vi "Resolve Header.vi"(6 "Metadata":variant, 8 "error in (no error)":errorcluster, 11 "CubeLogger in":refnum<class "CubeLogger.lvclass">) -> (0 "error out":errorcluster, 3 "CubeLogger out":refnum<class "CubeLogger.lvclass">)   [LabVIEW 2018, in "CubeLogger.lvclass"]
uses:
  CubeLogger.lvclass
  Header.ctl
  CubeLogger.lvclass/CubeLogger.ctl
panel:
  out "Canceled?":bool
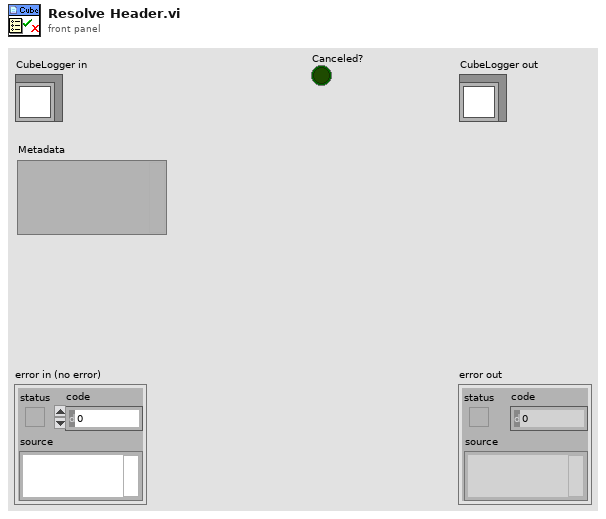
[diagram p1: front panel]
types:
  T1 = typedef "CubeLogger.lvclass/Header.ctl" = cluster{"name":string, "desc":string, "data":variant[], "meta":variant}
  T2 = enum16{"open", "replace", "create", "open or create", "replace or create", "replace or create with confirmation"}
  T3 = typedef "CubeLogger.lvclass/Dataset.ctl" = cluster{"name":string, "path":string, "size":i32[], "type":enum16{"single", "double", "uint8", "uint16", "uint32", "uint64", "int8", "int16", "int32", "int64"}, "mfmt":string}
  T4 = enum16{"single", "double", "uint8", "uint16", "uint32", "uint64", "int8", "int16", "int32", "int64"}
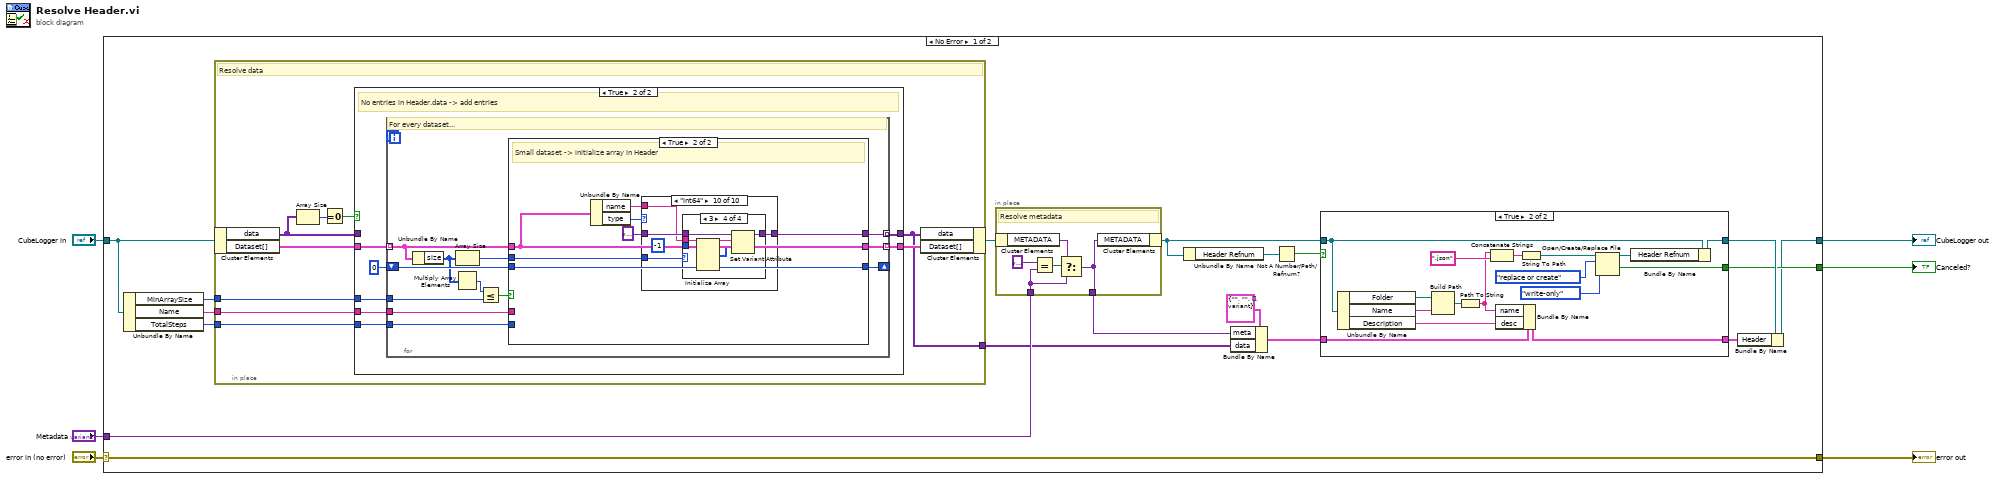
[diagram p0: block diagram]
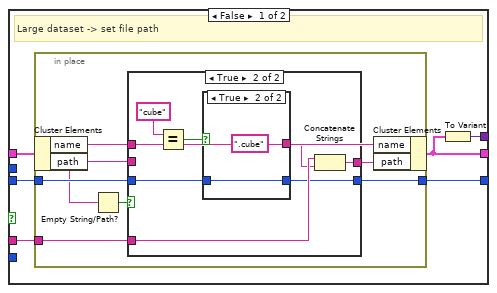
[diagram p4: hidden frame]
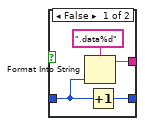
[diagram p6: hidden frame]
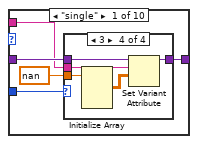
[diagram p7: hidden frame]
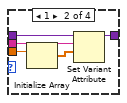
[diagram p9: hidden frame]
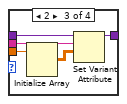
[diagram p10: hidden frame]
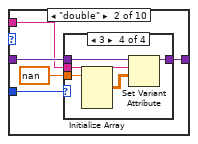
[diagram p11: hidden frame]
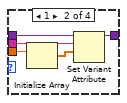
[diagram p13: hidden frame]
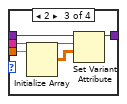
[diagram p14: hidden frame]
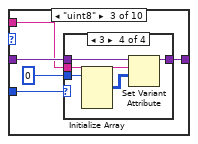
[diagram p15: hidden frame]
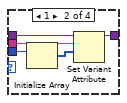
[diagram p17: hidden frame]
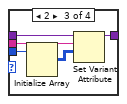
[diagram p18: hidden frame]
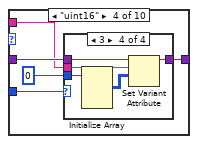
[diagram p19: hidden frame]
diagram:
  n1 = case shown="No Error" "error in (no error)" {
    selector: "error in (no error)" -> [w21 w326]
    tunnel: [w21 w326] -> w5
    tunnel: [w8 w325] -> w3
    tunnel: "CubeLogger in" -> [w23 w325]
    tunnel: "Metadata" -> [w24 _]
    tunnel: [w9 TRUE] -> w1
    frame No Error {
      n2 = Unbundle By Name(w23) -> ("MinArraySize"=w20:i32, "Name"=w19:string, "TotalSteps"=w18:i32)
      n3 = in-place {
        in-place-border: w20 -> [w49]
        in-place-border: w19 -> [w48]
        in-place-border: w18 -> [w47]
        in-place-border: [w46] -> w12
        # "Resolve data"
        n4 = in-place-cluster #1(w23) -> ("data"=w45:variant[], "Dataset[]"=w51:T3[])
        n5 = Array Size(array=w45) -> (size(s)=w44:i32)
        n6 = Equal To 0?(x=w44) -> (x = 0?=w43:bool)
        n7 = case shown="True" w43 {
          tunnel: w51 -> [w52 w60]
          tunnel: [w52 w59] -> w50
          tunnel: w49 -> [_ w58]
          tunnel: w45 -> [w53 _]
          tunnel: w48 -> [_ w57]
          tunnel: w47 -> [_ w56]
          tunnel: [w53 w55] -> w46
          frame False {
            # "Maybe: double check that everything is all right?\n   ... or not ..."
            # "Header.data has already been resolved -> do nothing"
          }
          frame True {
            # "No entries in Header.data -> add entries"
            n8 = for {
              tunnel: w60 -> [w72] mode=indexing
              shift-right: [w67] -> _
              shift-left: 0 -> [w68]
              tunnel: [w71] -> w59 mode=indexing
              tunnel: w57 -> [w69]
              tunnel: w58 -> [w70]
              tunnel: [w66] -> w55 mode=indexing
              tunnel: w56 -> [w65]
              # "For every dataset..."
              n9 = Unbundle By Name(w72) -> ("size"=w62:i32[])
              n10 = Multiply Array Elements(1:w62) -> (0:w64:i32)
              n11 = Array Size(array=w62) -> (size(s)=w61:i32)
              n12 = Less Or Equal?(x=w64, y=w70) -> (x <= y?=w63:bool)
              n13 = case shown="True" w63 {
                tunnel: [w73 w107] -> w71
                tunnel: w72 -> [w78 w107]
                tunnel: w69 -> [w77 _]
                tunnel: w68 -> [w76 w108]
                tunnel: [w75 w108] -> w67
                tunnel: [w74 w104] -> w66
                tunnel: w65 -> [_ _]
                tunnel: w61 -> [_ w102]
                frame False {
                  # "Large dataset -> set file path"
                  n14 = in-place {
                    in-place-border: w77 -> [w84]
                    in-place-border: w76 -> [w82]
                    in-place-border: [w81] -> w75
                    n15 = in-place-cluster #2(w78) -> ("name"=w79:string, "path"=w80:string)
                    n16 = Empty String/Path?(string/path=w80) -> (empty?=w85:bool)
                    n17 = case shown="True" w85 {
                      tunnel: w79 -> [_ w95]
                      tunnel: w84 -> [_ w91]
                      tunnel: [w87 w92] -> w83
                      tunnel: w82 -> [w86 w90]
                      tunnel: [w86 w89] -> w81
                      tunnel: w80 -> [w87 _]
                      frame False {
                      }
                      frame True {
                        n18 = Equal?(x="cube", y=w95) -> (x = y?=w93:bool)
                        n19 = case shown="True" w93 {
                          tunnel: w90 -> [w98 w101]
                          tunnel: [w97 w101] -> w89
                          tunnel: [w96 ".cube"] -> w88
                          frame False {
                            n20 = Format Into String(format string=".data%d", w98) -> (resulting string=w96:string)  [unwired: 2 in, 1 out]
                            n21 = Increment(x=w98) -> (x+1=w97:i32)
                          }
                          frame True {
                          }
                        }
                        n22 = Concatenate Strings(w91, w88) -> (w92:string)
                      }
                    }
                    n23 = in-place-cluster #2("name"=w79, "path"=w83) -> (w73:T3)
                  }
                  n24 = To Variant(anything=w73) -> (Variant=w74:variant)
                }
                frame True {
                  # "Small dataset -> initialize array in Header"
                  n25 = Unbundle By Name(w107) -> ("name"=w105:string, "type"=w106:T4)
                  n26 = case shown="\"int64\"" w106 {
                    tunnel: variant -> [w113 w134 w155 w176 w197 w218 w239 w260 w281 w302]
                    tunnel: w105 -> [w112 w133 w154 w175 w196 w217 w238 w259 w280 w301]
                    tunnel: [w111 w132 w153 w174 w195 w216 w237 w258 w279 w300] -> w104
                    tunnel: w102 -> [w110 w131 w152 w173 w194 w215 w236 w257 w278 w299]
                    frame "single" {
                      n27 = case shown="3" w110 {
                        tunnel: w113 -> [w114 w119 w124 w129]
                        tunnel: w112 -> [_ w118 w123 w128]
                        tunnel: [w114 w117 w122 w127] -> w111
                        tunnel: sgl nan -> [_ w116 w121 w126]
                        frame Default {
                        }
                        frame 1 {
                          n28 = Initialize Array(w116) -> (w115:sgl[])  [unwired: 1 in]
                          n29 = Set Variant Attribute(Variant=w119, name=w118, value=w115) -> (Variant out=w117:variant)  [unwired: 1 in, 2 out]
                        }
                        frame 2 {
                          n30 = Initialize Array(w121) -> (w120:sgl[][])  [unwired: 2 in]
                          n31 = Set Variant Attribute(Variant=w124, name=w123, value=w120) -> (Variant out=w122:variant)  [unwired: 1 in, 2 out]
                        }
                        frame 3 {
                          n32 = Initialize Array(w126) -> (w125:sgl[][][])  [unwired: 3 in]
                          n33 = Set Variant Attribute(Variant=w129, name=w128, value=w125) -> (Variant out=w127:variant)  [unwired: 1 in, 2 out]
                        }
                      }
                    }
                    frame "double" {
                      n34 = case shown="3" w131 {
                        tunnel: w134 -> [w135 w140 w145 w150]
                        tunnel: w133 -> [_ w139 w144 w149]
                        tunnel: [w135 w138 w143 w148] -> w132
                        tunnel: nan -> [_ w137 w142 w147]
                        frame Default {
                        }
                        frame 1 {
                          n35 = Initialize Array(w137) -> (w136:dbl[])  [unwired: 1 in]
                          n36 = Set Variant Attribute(Variant=w140, name=w139, value=w136) -> (Variant out=w138:variant)  [unwired: 1 in, 2 out]
                        }
                        frame 2 {
                          n37 = Initialize Array(w142) -> (w141:dbl[][])  [unwired: 2 in]
                          n38 = Set Variant Attribute(Variant=w145, name=w144, value=w141) -> (Variant out=w143:variant)  [unwired: 1 in, 2 out]
                        }
                        frame 3 {
                          n39 = Initialize Array(w147) -> (w146:dbl[][][])  [unwired: 3 in]
                          n40 = Set Variant Attribute(Variant=w150, name=w149, value=w146) -> (Variant out=w148:variant)  [unwired: 1 in, 2 out]
                        }
                      }
                    }
                    frame "uint8" {
                      n41 = case shown="3" w152 {
                        tunnel: w155 -> [w156 w161 w166 w171]
                        tunnel: w154 -> [_ w160 w165 w170]
                        tunnel: [w156 w159 w164 w169] -> w153
                        tunnel: u8 0 -> [_ w158 w163 w168]
                        frame Default {
                        }
                        frame 1 {
                          n42 = Initialize Array(w158) -> (w157:u8[])  [unwired: 1 in]
                          n43 = Set Variant Attribute(Variant=w161, name=w160, value=w157) -> (Variant out=w159:variant)  [unwired: 1 in, 2 out]
                        }
                        frame 2 {
                          n44 = Initialize Array(w163) -> (w162:u8[][])  [unwired: 2 in]
                          n45 = Set Variant Attribute(Variant=w166, name=w165, value=w162) -> (Variant out=w164:variant)  [unwired: 1 in, 2 out]
                        }
                        frame 3 {
                          n46 = Initialize Array(w168) -> (w167:u8[][][])  [unwired: 3 in]
                          n47 = Set Variant Attribute(Variant=w171, name=w170, value=w167) -> (Variant out=w169:variant)  [unwired: 1 in, 2 out]
                        }
                      }
                    }
                    frame "uint16" {
                      n48 = case shown="3" w173 {
                        tunnel: w176 -> [w177 w182 w187 w192]
                        tunnel: w175 -> [_ w181 w186 w191]
                        tunnel: [w177 w180 w185 w190] -> w174
                        tunnel: u16 0 -> [_ w179 w184 w189]
                        frame Default {
                        }
                        frame 1 {
                          n49 = Initialize Array(w179) -> (w178:u16[])  [unwired: 1 in]
                          n50 = Set Variant Attribute(Variant=w182, name=w181, value=w178) -> (Variant out=w180:variant)  [unwired: 1 in, 2 out]
                        }
                        frame 2 {
                          n51 = Initialize Array(w184) -> (w183:u16[][])  [unwired: 2 in]
                          n52 = Set Variant Attribute(Variant=w187, name=w186, value=w183) -> (Variant out=w185:variant)  [unwired: 1 in, 2 out]
                        }
                        frame 3 {
                          n53 = Initialize Array(w189) -> (w188:u16[][][])  [unwired: 3 in]
                          n54 = Set Variant Attribute(Variant=w192, name=w191, value=w188) -> (Variant out=w190:variant)  [unwired: 1 in, 2 out]
                        }
                      }
                    }
                    frame "uint32" {
                      n55 = case shown="3" w194 {
                        tunnel: w197 -> [w198 w203 w208 w213]
                        tunnel: w196 -> [_ w202 w207 w212]
                        tunnel: [w198 w201 w206 w211] -> w195
                        tunnel: u32 0 -> [_ w200 w205 w210]
                        frame Default {
                        }
                        frame 1 {
                          n56 = Initialize Array(w200) -> (w199:u32[])  [unwired: 1 in]
                          n57 = Set Variant Attribute(Variant=w203, name=w202, value=w199) -> (Variant out=w201:variant)  [unwired: 1 in, 2 out]
                        }
                        frame 2 {
                          n58 = Initialize Array(w205) -> (w204:u32[][])  [unwired: 2 in]
                          n59 = Set Variant Attribute(Variant=w208, name=w207, value=w204) -> (Variant out=w206:variant)  [unwired: 1 in, 2 out]
                        }
                        frame 3 {
                          n60 = Initialize Array(w210) -> (w209:u32[][][])  [unwired: 3 in]
                          n61 = Set Variant Attribute(Variant=w213, name=w212, value=w209) -> (Variant out=w211:variant)  [unwired: 1 in, 2 out]
                        }
                      }
                    }
                    frame "uint64" {
                      n62 = case shown="3" w215 {
                        tunnel: w218 -> [w219 w224 w229 w234]
                        tunnel: w217 -> [_ w223 w228 w233]
                        tunnel: [w219 w222 w227 w232] -> w216
                        tunnel: u64 0 -> [_ w221 w226 w231]
                        frame Default {
                        }
                        frame 1 {
                          n63 = Initialize Array(w221) -> (w220:u64[])  [unwired: 1 in]
                          n64 = Set Variant Attribute(Variant=w224, name=w223, value=w220) -> (Variant out=w222:variant)  [unwired: 1 in, 2 out]
                        }
                        frame 2 {
                          n65 = Initialize Array(w226) -> (w225:u64[][])  [unwired: 2 in]
                          n66 = Set Variant Attribute(Variant=w229, name=w228, value=w225) -> (Variant out=w227:variant)  [unwired: 1 in, 2 out]
                        }
                        frame 3 {
                          n67 = Initialize Array(w231) -> (w230:u64[][][])  [unwired: 3 in]
                          n68 = Set Variant Attribute(Variant=w234, name=w233, value=w230) -> (Variant out=w232:variant)  [unwired: 1 in, 2 out]
                        }
                      }
                    }
                    frame "int8" {
                      n69 = case shown="3" w236 {
                        tunnel: w239 -> [w240 w245 w250 w255]
                        tunnel: w238 -> [_ w244 w249 w254]
                        tunnel: [w240 w243 w248 w253] -> w237
                        tunnel: i8 -1 -> [_ w242 w247 w252]
                        frame Default {
                        }
                        frame 1 {
                          n70 = Initialize Array(w242) -> (w241:i8[])  [unwired: 1 in]
                          n71 = Set Variant Attribute(Variant=w245, name=w244, value=w241) -> (Variant out=w243:variant)  [unwired: 1 in, 2 out]
                        }
                        frame 2 {
                          n72 = Initialize Array(w247) -> (w246:i8[][])  [unwired: 2 in]
                          n73 = Set Variant Attribute(Variant=w250, name=w249, value=w246) -> (Variant out=w248:variant)  [unwired: 1 in, 2 out]
                        }
                        frame 3 {
                          n74 = Initialize Array(w252) -> (w251:i8[][][])  [unwired: 3 in]
                          n75 = Set Variant Attribute(Variant=w255, name=w254, value=w251) -> (Variant out=w253:variant)  [unwired: 1 in, 2 out]
                        }
                      }
                    }
                    frame "int16" {
                      n76 = case shown="3" w257 {
                        tunnel: w260 -> [w261 w266 w271 w276]
                        tunnel: w259 -> [_ w265 w270 w275]
                        tunnel: [w261 w264 w269 w274] -> w258
                        tunnel: i16 -1 -> [_ w263 w268 w273]
                        frame Default {
                        }
                        frame 1 {
                          n77 = Initialize Array(w263) -> (w262:i16[])  [unwired: 1 in]
                          n78 = Set Variant Attribute(Variant=w266, name=w265, value=w262) -> (Variant out=w264:variant)  [unwired: 1 in, 2 out]
                        }
                        frame 2 {
                          n79 = Initialize Array(w268) -> (w267:i16[][])  [unwired: 2 in]
                          n80 = Set Variant Attribute(Variant=w271, name=w270, value=w267) -> (Variant out=w269:variant)  [unwired: 1 in, 2 out]
                        }
                        frame 3 {
                          n81 = Initialize Array(w273) -> (w272:i16[][][])  [unwired: 3 in]
                          n82 = Set Variant Attribute(Variant=w276, name=w275, value=w272) -> (Variant out=w274:variant)  [unwired: 1 in, 2 out]
                        }
                      }
                    }
                    frame "int32" {
                      n83 = case shown="3" w278 {
                        tunnel: w281 -> [w282 w287 w292 w297]
                        tunnel: w280 -> [_ w286 w291 w296]
                        tunnel: [w282 w285 w290 w295] -> w279
                        tunnel: -1 -> [_ w284 w289 w294]
                        frame Default {
                        }
                        frame 1 {
                          n84 = Initialize Array(w284) -> (w283:i32[])  [unwired: 1 in]
                          n85 = Set Variant Attribute(Variant=w287, name=w286, value=w283) -> (Variant out=w285:variant)  [unwired: 1 in, 2 out]
                        }
                        frame 2 {
                          n86 = Initialize Array(w289) -> (w288:i32[][])  [unwired: 2 in]
                          n87 = Set Variant Attribute(Variant=w292, name=w291, value=w288) -> (Variant out=w290:variant)  [unwired: 1 in, 2 out]
                        }
                        frame 3 {
                          n88 = Initialize Array(w294) -> (w293:i32[][][])  [unwired: 3 in]
                          n89 = Set Variant Attribute(Variant=w297, name=w296, value=w293) -> (Variant out=w295:variant)  [unwired: 1 in, 2 out]
                        }
                      }
                    }
                    frame "int64" {
                      n90 = case shown="3" w299 {
                        tunnel: w302 -> [w303 w308 w313 w318]
                        tunnel: w301 -> [_ w307 w312 w317]
                        tunnel: [w303 w306 w311 w316] -> w300
                        tunnel: i64 -1 -> [_ w305 w310 w315]
                        frame Default {
                        }
                        frame 1 {
                          n91 = Initialize Array(w305) -> (w304:i64[])  [unwired: 1 in]
                          n92 = Set Variant Attribute(Variant=w308, name=w307, value=w304) -> (Variant out=w306:variant)  [unwired: 1 in, 2 out]
                        }
                        frame 2 {
                          n93 = Initialize Array(w310) -> (w309:i64[][])  [unwired: 2 in]
                          n94 = Set Variant Attribute(Variant=w313, name=w312, value=w309) -> (Variant out=w311:variant)  [unwired: 1 in, 2 out]
                        }
                        frame 3 {
                          n95 = Initialize Array(w315) -> (w314:i64[][][])  [unwired: 3 in]
                          n96 = Set Variant Attribute(Variant=w318, name=w317, value=w314) -> (Variant out=w316:variant)  [unwired: 1 in, 2 out]
                        }
                      }
                    }
                  }
                }
              }
            }
          }
        }
        n97 = in-place-cluster #1("data"=w46, "Dataset[]"=w50) -> (w22:refnum<class "CubeLogger.lvclass">)
      }
      n98 = in-place {
        in-place-border: w24 -> [w320]
        in-place-border: [w322] -> w14
        # "Resolve metadata"
        n99 = in-place-cluster #3(w22) -> ("METADATA"=w323:variant)
        n100 = Equal?(x=variant, y=w320) -> (x = y?=w319:bool)
        n101 = Select(t=w323, s=w319, f=w320) -> (s? t:f=w322:variant)
        n102 = in-place-cluster #3("METADATA"=w322) -> (w16:refnum<class "CubeLogger.lvclass">)
      }
      n103 = Unbundle By Name(w16) -> ("Header Refnum"=w10:refnum<file>)
      n104 = Bundle By Name(cluster=T1 {"name"="", "desc"="", "data"=[], "meta"=variant} ("Header"), "meta"=w14, "data"=w12) -> (w11:T1)
      n105 = Not A Number/Path/Refnum?(number/path/refnum=w10) -> (NaN/Path/Refnum?=w15:bool)
      n106 = case shown="True" w15 {
        tunnel: [w25 w38] -> w7
        tunnel: [w26 w28] -> w17
        tunnel: w16 -> [w26 w37]
        tunnel: w11 -> [w25 w36]
        tunnel: [_ w29] -> w9
        frame False {
        }
        frame True {
          n107 = Unbundle By Name(w37) -> ("Folder"=w41:path, "Name"=w42:string, "Description"=w39:string)
          n108 = Build Path(base path=w41, name or relative path=w42) -> (appended path=w40:path)
          n109 = Path To String(path=w40) -> (string=w34:string)
          n110 = Concatenate Strings(w34, ".json" ("string")) -> (w33:string)
          n111 = Bundle By Name(cluster=w36, "name"=w34, "desc"=w39) -> (w38:T1)
          n112 = String To Path(string=w33) -> (path=w32:path)
          n113 = Open/Create/Replace File(file path (use dialog)=w32, operation (0:open)=T2."replace or create", access (0:read/write)=enum16{"read/write", "read-only", "write-only"}."write-only") -> (refnum out=w27:refnum<file>, cancelled=w29:bool)  [unwired: 3 in, 1 out]
          n114 = Bundle By Name(cluster=w37, "Header Refnum"=w27) -> (w28:refnum<class "CubeLogger.lvclass">)
        }
      }
      n115 = Bundle By Name(cluster=w17, "Header"=w7) -> (w8:refnum<class "CubeLogger.lvclass">)
    }
    frame Error {
    }
  }
  "error out" <- w5
  "CubeLogger out" <- w3
  "Canceled?" <- w1
